vi "Check Installed.vi"(8 "error in (no error)":errorcluster, 11 "TestStand Adapter in":refnum<class "TestStand Adapter.lvclass">) -> (0 "error out":errorcluster, 1 "Version":string, 2 "Installed?":bool, 3 "TestStand Adapter out":refnum<class "TestStand Adapter.lvclass">)   [LabVIEW 2026, in "TestStand Adapter.lvclass"]
uses:
  TestStand Adapter.lvclass
  TestStand Adapter.lvclass/TestStand Adapter.ctl
  <vilib>/regexp/Match Regular Expression.xnode
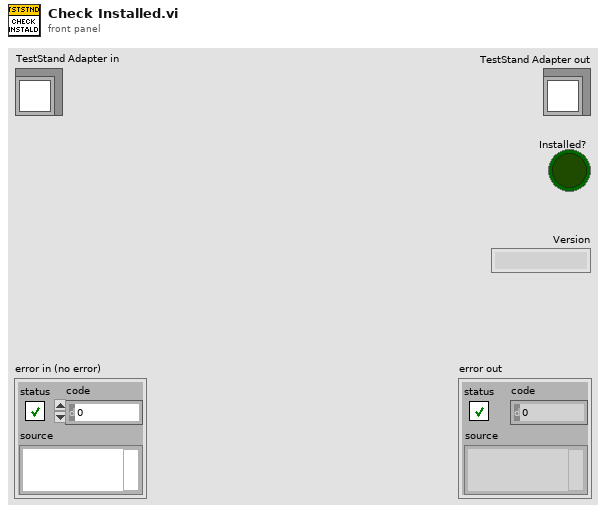
[diagram p1: front panel]
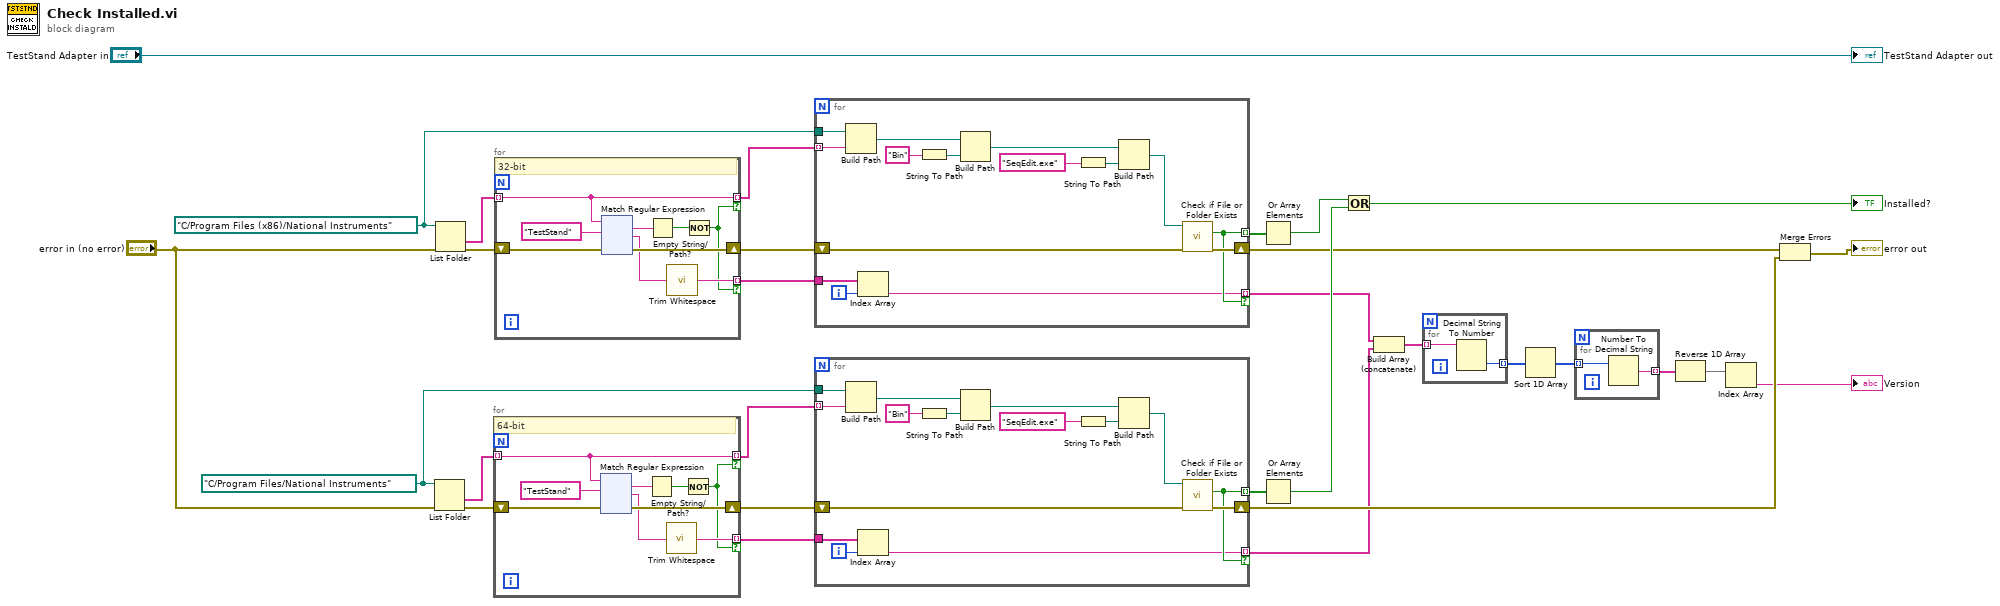
[diagram p0: block diagram]
diagram:
  w17 = path "C:/Program Files/National Instruments" ("path")
  w23 = path "C:/Program Files (x86)/National Instruments" ("path")
  n1 = List Folder(path=w17, error in="error in (no error)") -> (folder names=w26:string[], error out=w27:errorcluster)  [unwired: 2 in, 2 out]
  n2 = List Folder(path=w23, error in="error in (no error)") -> (folder names=w29:string[], error out=w28:errorcluster)  [unwired: 2 in, 2 out]
  n3 = for {
    tunnel: w26 -> [w34] mode=indexing
    shift-right: [w35] -> w19
    shift-left: w27 -> [w39]
    tunnel: [w34] -> w18 mode=indexing if=w31
    tunnel: [w32] -> w16 mode=indexing if=w31
    # "64-bit"
    n4 = xnode "Match Regular Expression"("input string"=w34, "regular expression"="TestStand", "error in"=w39) -> ("whole match"=w37:string, "after match"=w33:string, "error out"=w35:errorcluster)  [unwired: 3 in, 2 out]
    n5 = Empty String/Path?(string/path=w37) -> (empty?=w36:bool)
    n6 = call <vilib>:"Trim Whitespace.vi"("string"=w33) -> ("trimmed string"=w32:string)  [unwired: 1 in]
    n7 = Not(x=w36) -> (.not. x?=w31:bool)
  }
  n8 = for {
    tunnel: w29 -> [w160] mode=indexing
    shift-right: [w161] -> w21
    shift-left: w28 -> [w165]
    tunnel: [w160] -> w22 mode=indexing if=w157
    tunnel: [w158] -> w20 mode=indexing if=w157
    # "32-bit"
    n9 = xnode "Match Regular Expression"("input string"=w160, "regular expression"="TestStand", "error in"=w165) -> ("whole match"=w163:string, "after match"=w159:string, "error out"=w161:errorcluster)  [unwired: 3 in, 2 out]
    n10 = Empty String/Path?(string/path=w163) -> (empty?=w162:bool)
    n11 = call <vilib>:"Trim Whitespace.vi"("string"=w159) -> ("trimmed string"=w158:string)  [unwired: 1 in]
    n12 = Not(x=w162) -> (.not. x?=w157:bool)
  }
  n13 = for {
    tunnel: w23 -> [w297]
    tunnel: w22 -> [w296] mode=indexing
    shift-right: [w287] -> w11
    shift-left: w21 -> [w288]
    tunnel: [w286] -> w15 mode=indexing
    tunnel: [w283] -> w8 mode=indexing if=w286
    tunnel: w20 -> [w285]
    i -> [w284]
    n14 = Build Path(base path=w297, name or relative path=w296) -> (appended path=w295:path)
    n15 = Index Array(array=w285, index=w284) -> (element=w283:string)
    n16 = String To Path(string="Bin") -> (path=w293:path)
    n17 = Build Path(base path=w295, name or relative path=w293) -> (appended path=w290:path)
    n18 = String To Path(string="SeqEdit.exe") -> (path=w292:path)
    n19 = Build Path(base path=w290, name or relative path=w292) -> (appended path=w289:path)
    n20 = call <vilib>:"Check if File or Folder Exists.vi"("error in (no error)"=w288, "path"=w289) -> ("error out"=w287:errorcluster, "file or folder exists?"=w286:bool)  [unwired: 7 in, 1 out]
  }
  n21 = for {
    tunnel: w17 -> [w312]
    tunnel: w18 -> [w311] mode=indexing
    shift-right: [w302] -> w9
    shift-left: w19 -> [w303]
    tunnel: [w301] -> w14 mode=indexing
    tunnel: [w298] -> w7 mode=indexing if=w301
    tunnel: w16 -> [w300]
    i -> [w299]
    n22 = Build Path(base path=w312, name or relative path=w311) -> (appended path=w310:path)
    n23 = Index Array(array=w300, index=w299) -> (element=w298:string)
    n24 = String To Path(string="Bin") -> (path=w308:path)
    n25 = Build Path(base path=w310, name or relative path=w308) -> (appended path=w305:path)
    n26 = String To Path(string="SeqEdit.exe") -> (path=w307:path)
    n27 = Build Path(base path=w305, name or relative path=w307) -> (appended path=w304:path)
    n28 = call <vilib>:"Check if File or Folder Exists.vi"("error in (no error)"=w303, "path"=w304) -> ("error out"=w302:errorcluster, "file or folder exists?"=w301:bool)  [unwired: 7 in, 1 out]
  }
  n29 = Or Array Elements(Boolean array=w15) -> (logical OR=w13:bool)
  n30 = Or Array Elements(Boolean array=w14) -> (logical OR=w12:bool)
  n31 = Or(x=w13, y=w12) -> (x .or. y?=→"Installed?":bool)
  n32 = Build Array (concatenate)(w8, w7) -> (w6:string[])
  n33 = for {
    tunnel: w6 -> [w314] mode=indexing
    tunnel: [w313] -> w5 mode=indexing
    n34 = Decimal String To Number(string=w314) -> (number=w313:i32)  [unwired: 2 in, 1 out]
  }
  n35 = Sort 1D Array(array=w5) -> (sorted array=w4:i32[])
  n36 = for {
    tunnel: w4 -> [w316] mode=indexing
    tunnel: [w315] -> w3 mode=indexing
    n37 = Number To Decimal String(number=w316) -> (decimal integer string=w315:string)  [unwired: 1 in]
  }
  n38 = Reverse 1D Array(array=w3) -> (reversed array=w2:string[])
  n39 = Index Array(array=w2) -> (element=→"Version":string)  [unwired: 1 in]
  n40 = Merge Errors(w11, w9) -> (→"error out":errorcluster)
  "TestStand Adapter out" <- "TestStand Adapter in"
